vi "Start.vi"(8 "error in (no error)":errorcluster, 11 "number of modules":i16) -> (0 "error out":errorcluster)   [LabVIEW 2017, in "MCSA_9065_API.lvlib"]
uses:
  <vilib>/addons/InsightCM/Devices/Shared/Mcsa/Fpga/McsaAcquire/subVIs/McsaAPI_9065/MCSA_9065_API.lvlib
  <vilib>/eio/EIONode/EIONode.xnode
  <vilib>/rvi/eio/common/nirviEmuTemplateMethod_errors.vi
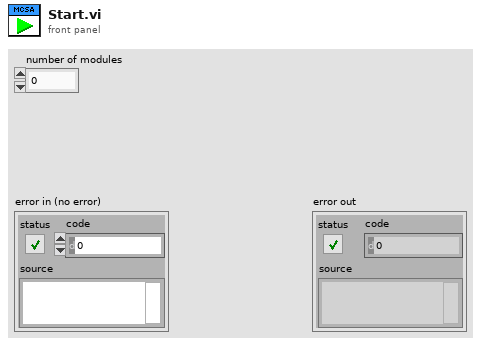
[diagram p1: front panel]
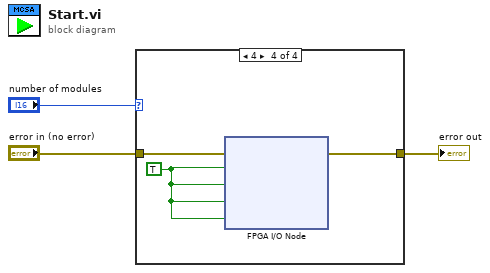
[diagram p0: block diagram]
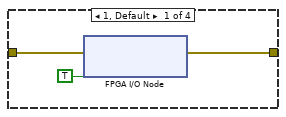
[diagram p2: hidden frame]
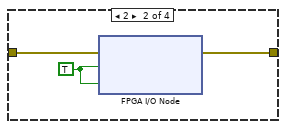
[diagram p3: hidden frame]
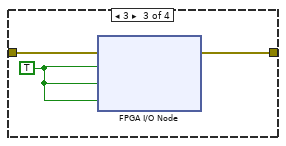
[diagram p4: hidden frame]
diagram:
  n1 = case shown="4" "number of modules" {
    tunnel: "error in (no error)" -> [w5 w8 w12 w15]
    tunnel: [w6 w9 w10 w14] -> w1
    frame 1, Default {
      n2 = xnode "FPGA I/O Node"("error in"=w5, "Mod1/Start"=TRUE) -> ("error out"=w6:errorcluster)  [unwired: 1 in, 1 out]
    }
    frame 2 {
      w7 = TRUE
      n3 = xnode "FPGA I/O Node"("error in"=w8, "Mod1/Start"=w7, "Mod2/Start"=w7) -> ("error out"=w9:errorcluster)  [unwired: 2 in, 2 out]
    }
    frame 3 {
      w11 = TRUE ("Mod1/Start")
      n4 = xnode "FPGA I/O Node"("error in"=w12, "Mod1/Start"=w11, "Mod2/Start"=w11, "Mod3/Start"=w11) -> ("error out"=w10:errorcluster)  [unwired: 3 in, 3 out]
    }
    frame 4 {
      w13 = TRUE ("Mod1/Start")
      n5 = xnode "FPGA I/O Node"("error in"=w15, "Mod1/Start"=w13, "Mod2/Start"=w13, "Mod3/Start"=w13, "Mod4/Start"=w13) -> ("error out"=w14:errorcluster)  [unwired: 4 in, 4 out]
    }
  }
  "error out" <- w1
